vi "PC_create_unique_tdms_file.vi"(8 "error in (no error)":errorcluster, 9 "string":string, 10 "Recording Name":string, 11 "Experiment Folder":path) -> (0 "error out":errorcluster, 3 "Refnum out":refnum<k34>)   [LabVIEW 2020]
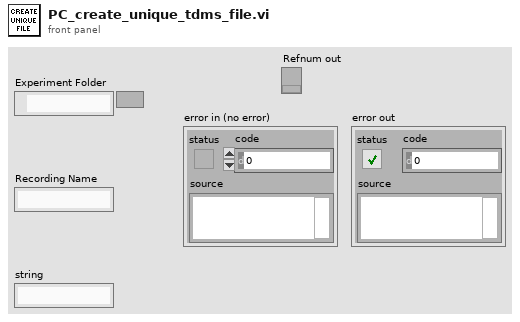
[diagram p1: front panel]
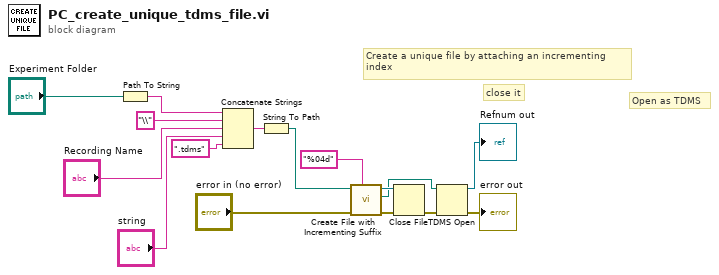
[diagram p0: block diagram]
diagram:
  # "Open as TDMS"
  # "close it"
  # "Create a unique file by attaching an incrementing \nindex"
  n1 = Path To String(path="Experiment Folder") -> (string=w3:string)
  n2 = Concatenate Strings(w3, "\\" ("string"), "Recording Name", "string", ".tdms" ("string")) -> (w5:string)
  n3 = String To Path(string=w5) -> (path=w8:path)
  n4 = call <vilib>:"Create File with Incrementing Suffix.vi"("format string (\" (%d)\")"="%04d" ("format string (\" (%d)\")"), "error in (no error)"="error in (no error)", "file path"=w8) -> ("error out"=w9:errorcluster, "actual path"=w7:path, "refnum out"=w10:refnum<file>)  [unwired: 6 in]
  n5 = Close File(refnum=w10, error in=w9) -> (error out=w11:errorcluster)  [unwired: 1 out]
  n6 = TDMS Open(8:w11, 11:w7) -> (0:→"error out":errorcluster, 3:→"Refnum out":refnum<k34>)  [unwired: 5 in]
